vi "DecodeBalls.vi"(8 "error in":errorcluster, 9 "array":u8[](array[numeric]), 10 "Key":i32=5) -> (0 "error out":errorcluster, 1 "array w/ subset deleted out":u8[](array[numeric]), 3 "ball":T1)   [LabVIEW 2017]
uses:
  Core/AI Ball.ctl
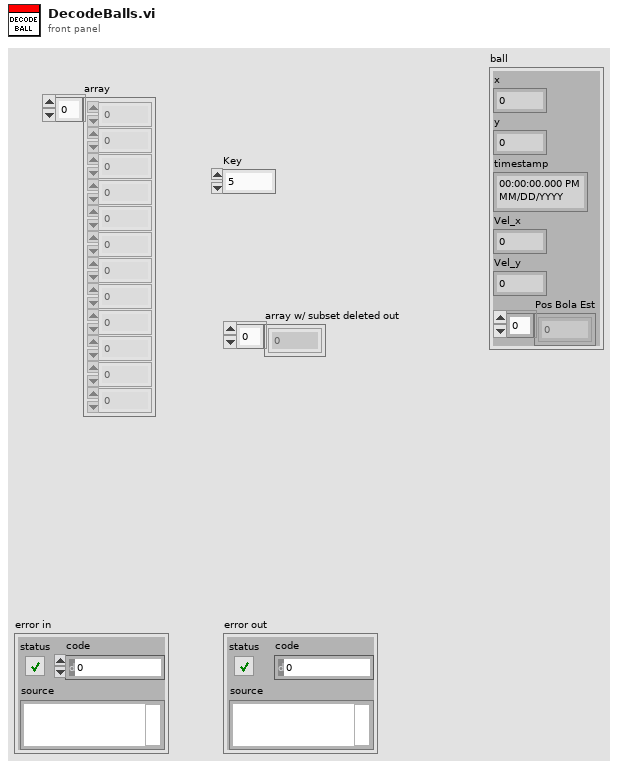
[diagram p1: front panel]
types:
  T1 = typedef "AI Ball.ctl" = cluster{"x":dbl, "y":dbl, "timestamp":timestamp, "Vel_x":dbl, "Vel_y":dbl, "Pos Bola Est":dbl[]}
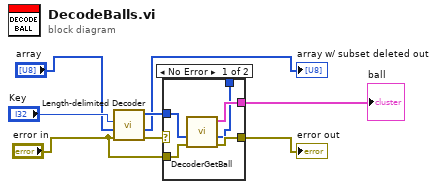
[diagram p0: block diagram]
diagram:
  n1 = call "Length-delimited Decoder.vi"("error in (no error)"="error in", "Array"="array", "Key"="Key") -> ("error out"=w4:errorcluster, "array w/ subset deleted"=→"array w/ subset deleted out":u8[], "Length-delimited"=w2:u8[])  [unwired: 5 in, 1 out]
  n2 = case shown="No Error" w4 {
    tunnel: [w11 w14] -> w8
    tunnel: w2 -> [w13 _]
    tunnel: "error in" -> [w12 w14]
    tunnel: [w10 _] -> w5
    tunnel: [w9 _] -> _
    frame No Error {
      n3 = call "DecoderGetBall.vi"("error in"=w12, "Array"=w13) -> ("error out"=w11:errorcluster, "array w/ subset deleted"=w9:u8[], "ball"=w10:T1)  [unwired: 7 in]
    }
    frame Error {
    }
  }
  "error out" <- w8
  "ball" <- w5
